vi "getColor.vi"(8 "error in (no error)":errorcluster) -> (0 "error out":errorcluster, 2 "ok":bool, 3 "Color":u32(colorbox))   [LabVIEW 2017, in "QControl_Graph.lvclass"]
uses:
  QControl_Graph.lvclass
  selectColor.vi
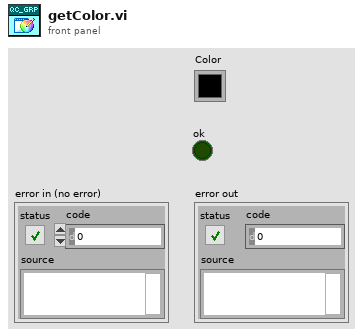
[diagram p1: front panel]
types:
  T1 = enum32{"Invalid", "Standard", "Closed", "Hidden", "Minimized", "Maximized"}
  T2 = enum32{"Invalid", "Default", "Floating", "Floating/Auto-Hide", "Modal"}
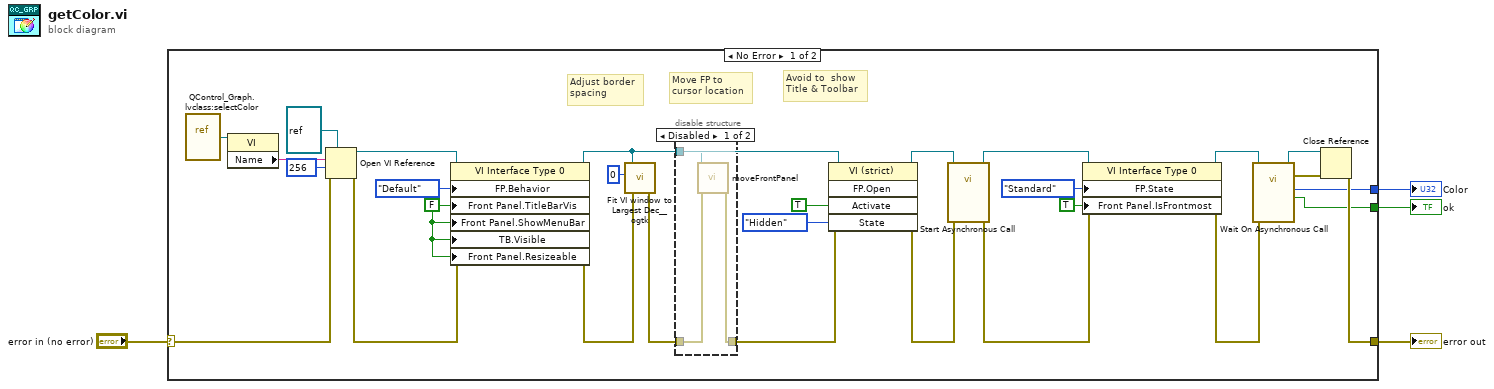
[diagram p0: block diagram]
diagram:
  n1 = case shown="No Error" "error in (no error)" {
    selector: "error in (no error)" -> [w12 w38]
    tunnel: [w11 w38] -> w3
    tunnel: [w10 _] -> w2
    tunnel: [w9 _] -> w1
    frame No Error {
      w32 = FALSE ("Front Panel Window:Title Bar Visible")
      # "Adjust border\nspacing"
      # "Move FP to \ncursor location"
      # "Avoid to  show\nTitle & Toolbar"
      n2 = vi-ref "QControl_Graph.lvclass:selectColor.vi"() -> (w26:refnum<vi>)
      n3 = property class="VI"(reference=w26) -> ("Name"=w25:string)  [unwired: 1 in, 2 out]
      n4 = Open VI Reference(type specifier VI Refnum (for type only)=refnum<vi> refnum, vi path=w25, options=256, error in (no error)=w12) -> (vi reference=w22:refnum<vi>, error out=w21:errorcluster)  [unwired: 2 in]
      n5 = property class="VI Interface Type 0"(reference=w22, error in=w21, "FP.Behavior"=T2."Default" ("Front Panel Window:Behavior"), "Front Panel.TitleBarVis"=w32, "Front Panel.ShowMenuBar"=w32, "TB.Visible"=w32, "Front Panel.Resizeable"=w32) -> (reference out=w5:refnum<vi>, error out=w7:errorcluster)
      n6 = call <userlib>:"Fit VI window to Largest Dec__ogtk.vi"("error in (no error)"=w7, "border spacing (2 px)"=0, "VI Ref (calling VI)"=w5) -> ("error out"=w6:errorcluster)  [unwired: 3 in, 1 out]
      n7 = disable-structure shown="Disabled" {
        disable-tunnel: [w36 w37] -> w28
        disable-tunnel: w6 -> [w35 w37]
        disable-tunnel: w5 -> [w34 _]
        frame Disabled {
          n8 = call "moveFrontPanel.vi"("error in (no error)"=w35, "VI in"=w34) -> ("error out"=w36:errorcluster)  [unwired: 8 in, 1 out]
        }
        frame Enabled {
        }
      }
      n9 = invoke class="VI (strict)" method="FP.Open"(reference=w5, error in=w28, "Activate"=TRUE ("Activate?"), "State"=T1."Hidden") -> (reference out=w20:refnum<vi>, error out=w18:errorcluster)  [unwired: 1 in, 3 out]
      n10 = call-by-ref "Start Asynchronous Call"(reference=w20, error in=w18) -> (reference out=w19:refnum<vi>, error out=w17:errorcluster)  [unwired: 10 in, 2 out]
      n11 = property class="VI Interface Type 0"(reference=w19, error in=w17, "FP.State"=T1."Standard" ("Front Panel Window:State"), "Front Panel.IsFrontmost"=TRUE ("Activate?")) -> (reference out=w16:refnum<vi>, error out=w15:errorcluster)
      n12 = call-by-ref "Wait On Asynchronous Call"(reference=w16, error in=w15) -> (reference out=w14:refnum<vi>, error out=w13:errorcluster, "ok"=w9:bool, 3:w10:u32)  [unwired: 10 in]
      n13 = Close Reference(reference=w14, error in (no error)=w13) -> (error out=w11:errorcluster)
    }
    frame Error {
    }
  }
  "error out" <- w3
  "Color" <- w2
  "ok" <- w1
